vi "MTS_PreapareImage.vi"(0 "WS File Tree":refnum<vi>, 5 "Workspace":path, 7 "Measurement Type":T3(ring), 9 "Image Measurent Parameters":T1, 11 "error in":errorcluster) -> (4 "File Name (dup)":path, 6 "File No":i32, 8 "Image Header":T2, 10 "Comment":string, 15 "error out":errorcluster)   [LabVIEW 2013]
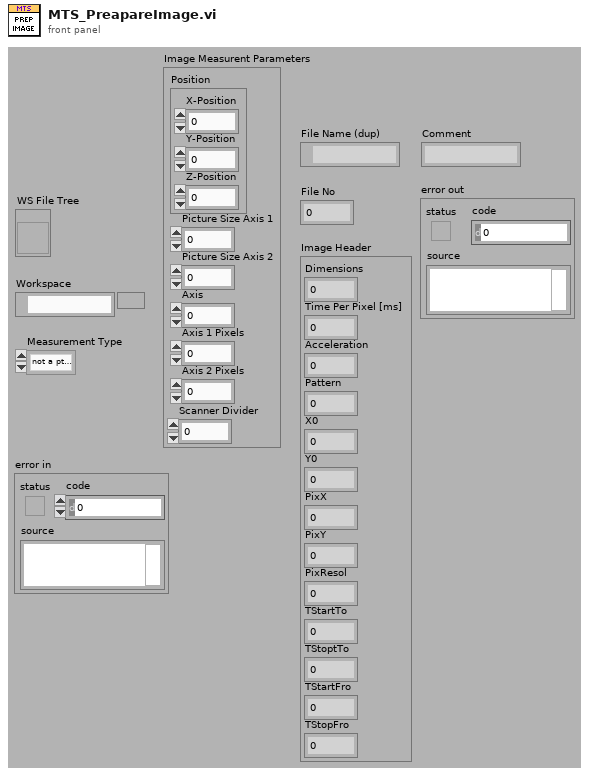
[diagram p1: front panel]
types:
  T1 = cluster{"Position":cluster{"X-Position":dbl, "Y-Position":dbl, "Z-Position":dbl}, "Picture Size Axis 1":dbl, "Picture Size Axis 2":dbl, "Axis":i32, "Axis 1 Pixels":u16, "Axis 2 Pixels":u16, "Scanner Divider":i32}
  T2 = cluster{"Dimensions":i32, "Time Per Pixel [ms]":dbl, "Acceleration":i32, "Pattern":i32, "X0":sgl, "Y0":sgl, "PixX":i32, "PixY":i32, "PixResol":sgl, "TStartTo":sgl, "TStoptTo":sgl, "TStartFro":sgl, "TStopFro":sgl}
  T3 = enum16{"not a pt3 File", "Image File", "Point Measurement", "Auto Point", "Line Scan"}
  T4 = enum16{"unknown", "pt3 File", "png Image", "bmp Image"}
  T5 = cluster{"X-Position":dbl, "Y-Position":dbl, "Z-Position":dbl}
  T6 = cluster{"Picture Size":dbl[], "Pixels":i32[], "Upper Left":cluster{"x-Position":dbl, "y-Position":dbl, "z-Position":dbl}}
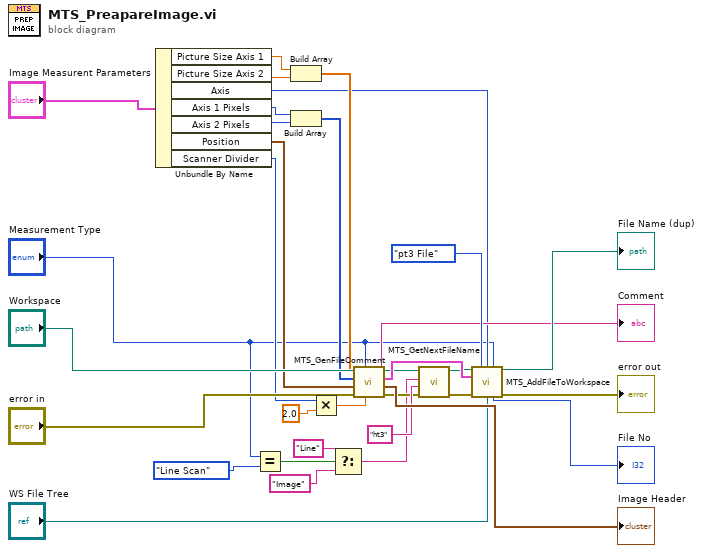
[diagram p0: block diagram]
diagram:
  n1 = Unbundle By Name("Image Measurent Parameters") -> ("Picture Size Axis 1"=w15:dbl, "Picture Size Axis 2"=w14:dbl, "Axis"=w7:i32, "Axis 1 Pixels"=w11:u16, "Axis 2 Pixels"=w12:u16, "Position"=w9:T5, "Scanner Divider"=w8:i32)
  n2 = Equal?(x="Measurement Type", y=T3."Line Scan" ("Measurement Type")) -> (x = y?=w4:bool)
  n3 = Build Array(w15, w14) -> (w13:dbl[])
  n4 = Build Array(w11, w12) -> (w10:u16[])
  n5 = Multiply(x=w8, y=2.0) -> (x*y=w30:dbl)
  n6 = Select(t="Line" ("Measurement Type"), s=w4, f="Image" ("Measurement Type")) -> (s? t:f=w3:string)
  n7 = call "MTS_GenFileComment.vi"("Time Per Pixel [ms]"=w30, "Measurement Type"="Measurement Type", "error in"="error in", "Upper Left"=w9, "Pixels"=w10, "Picture Size"=w13) -> ("error out"=w20:errorcluster, "Image Header"=→"Image Header":T2, "Image Info"=w25:T6, "Comment"=→"Comment":string)  [unwired: 2 in]
  n8 = call "MTS_GetNextFileName.vi"("error in (no error)"=w20, "File Type"="ht3", "Measurement Type"=w3, "Workspace"="Workspace") -> ("error out"=w22:errorcluster, "Next File Name"=w23:path)  [unwired: 6 in]
  n9 = call "MTS_AddFileToWorkspace.vi"("File Name"=w23, "File Type"=T4."pt3 File", "Scan Axis"=w7, "Measurement Type"="Measurement Type", "File Info"=w25, "error in (no error)"=w22, "Tree Refnum"="WS File Tree") -> ("File Name (dup)"=→"File Name (dup)":path, "File No"=→"File No":i32, "error out"=→"error out":errorcluster)  [unwired: 6 in]
